vi "rollingAverage_multi.vi"   [LabVIEW 2011]
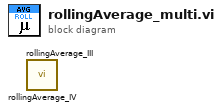
[diagram p0: block diagram]
diagram:
  n1 = call "rollingAverage_IV.vi"() -> ()  [unwired: 8 in, 4 out]
  n2 = call "rollingAverage_III.vi"() -> ()  [unwired: 9 in, 3 out]
